vi "Remove Team.vi"(8 "error in (no error)":errorcluster, 10 "Team":refnum<class "Team.lvclass">, 11 "Game in":refnum<class "Game.lvclass">) -> (0 "error out":errorcluster, 3 "Game out":refnum<class "Game.lvclass">)   [LabVIEW 2020, in "SquareBattle.lvlib" / "Game.lvclass"]
uses:
  Game.lvclass
  Team/Team.lvclass
  Game.lvclass/Game.ctl
  Team/Team.lvclass/Team.ctl
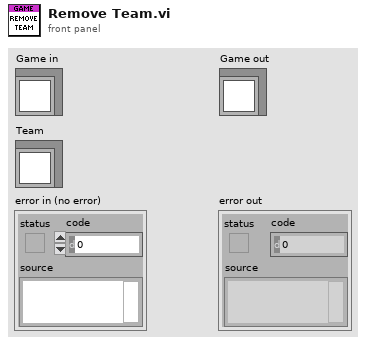
[diagram p1: front panel]
types:
  T1 = typedef "SquareBattle.lvlib/Team ID.ctl" = u32
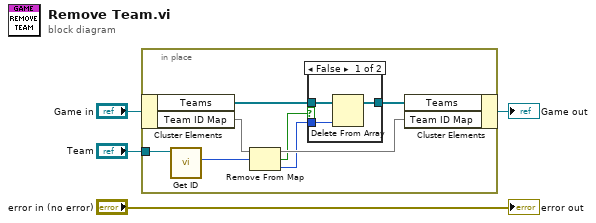
[diagram p0: block diagram]
diagram:
  n1 = in-place {
    in-place-border: "Team" -> [w12]
    n2 = in-place-cluster #1("Game in") -> ("Teams"=w6:refnum<class "Team.lvclass">[], "Team ID Map"=w11:map{T1, i32})
    n3 = call "Get ID.vi"("Team in"=w12) -> ("Team ID"=w10:T1)  [unwired: 10 in]
    n4 = Remove From Map(10:w10, 11:w11) -> (1:w7:i32, 2:w8:bool, 3:w9:map{T1, i32})
    n5 = case shown="False" w8 {
      tunnel: w7 -> [w14 _]
      tunnel: w6 -> [w15 w16]
      tunnel: [w13 w16] -> w5
      frame False {
        n6 = Delete From Array(array=w15, index=w14) -> (array with subset deleted=w13:refnum<class "Team.lvclass">[])  [unwired: 1 in, 1 out]
      }
      frame True {
      }
    }
    n7 = in-place-cluster #1("Teams"=w5, "Team ID Map"=w9) -> (→"Game out":refnum<class "Game.lvclass">)
  }
  "error out" <- "error in (no error)"
